vi "Intake Pistion LOgic.vi"(1 "Y Button":bool, 2 "X Button":bool) -> ()   [LabVIEW 2015]
uses:
  <vilib>/Rock Robotics/WPI/Solenoid/WPI_SolenoidValue.ctl
  <vilib>/Rock Robotics/WPI/Solenoid/WPI_SolenoidSetEnum.vi
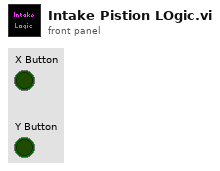
[diagram p1: front panel]
types:
  T1 = typedef "WPI_SolenoidDevRef.ctl" = cluster{"DevStatus":errorcluster, "Pneumatics Control Module":u8, "Forward Solenoid Channel":T2, "Reverse Solenoid Channel":T2}
  T2 = typedef "WPI_SolenoidChannel.ctl" = enum8{"Solenoid 0", "Solenoid 1", "Solenoid 2", "Solenoid 3", "Solenoid 4", "Solenoid 5", "Solenoid 6", "Solenoid 7", "Invalid"}
  T3 = typedef "WPI_SolenoidValue.ctl" = enum16{"Off", "On", "Forward", "Reverse"}
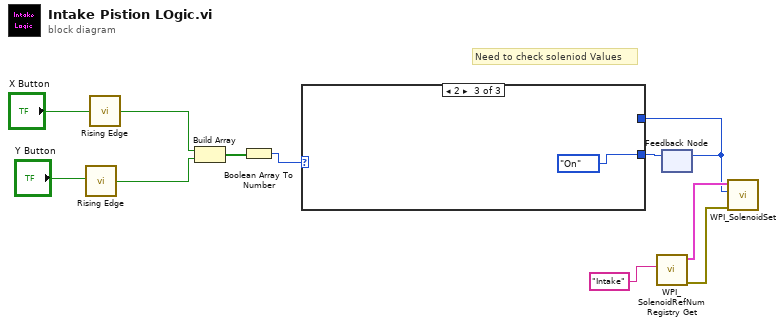
[diagram p0: block diagram]
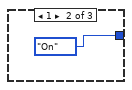
[diagram p3: hidden frame]
diagram:
  # "Need to check soleniod Values"
  n1 = call "Rising Edge.vi"("Button Pressed?"="Y Button") -> ("Bool Output"=w8:bool)
  n2 = call "Rising Edge.vi"("Button Pressed?"="X Button") -> ("Bool Output"=w9:bool)
  n3 = Build Array(w9, w8) -> (w7:bool[])
  n4 = Boolean Array To Number(Boolean array=w7) -> (number=w6:u32)
  n5 = call <vilib>:"WPI_SolenoidRefNum Registry Get.vi"("refnum name"="Intake") -> ("error out"=w4:errorcluster, "SolenoidDevRef"=w5:T1)  [unwired: 9 in]
  n6 = feedback #1() -> (w1:T3)  [unwired: 1 in]
  n7 = case shown="2" w6 {
    tunnel: [w12 WPI_SolenoidValue."On" ("Value") WPI_SolenoidValue."On" ("Value")] -> w2
    tunnel: w1 -> [w12 _ _]
    frame 0, Default {
    }
    frame 1 {
    }
    frame 2 {
    }
  }
  n8 = feedback-in #1(w2) -> ()
  n9 = call-poly <vilib>:"WPI_SolenoidSet.vi"("error in (no error)"=w4, "Value"=w1, "SolenoidDevRef"=w5) -> ()  [unwired: 7 in, 2 out]
